vi "NamesofPMUsElements.vi"(8 "DigitalNum":u8, 9 "AnalogNum":u8, 10 "PhasorsNum":u8, 11 "data in":string) -> (1 "Phasor Digitals":i32(listbox), 2 "PMU Analogs":i32(listbox), 3 "Phasor Names":i32(listbox))   [LabVIEW 2013]
panel:
  out "DIGUNIT":string
  out "ANUNIT":string
  out "PHUNIT":string
  out "RET_DATA":T1
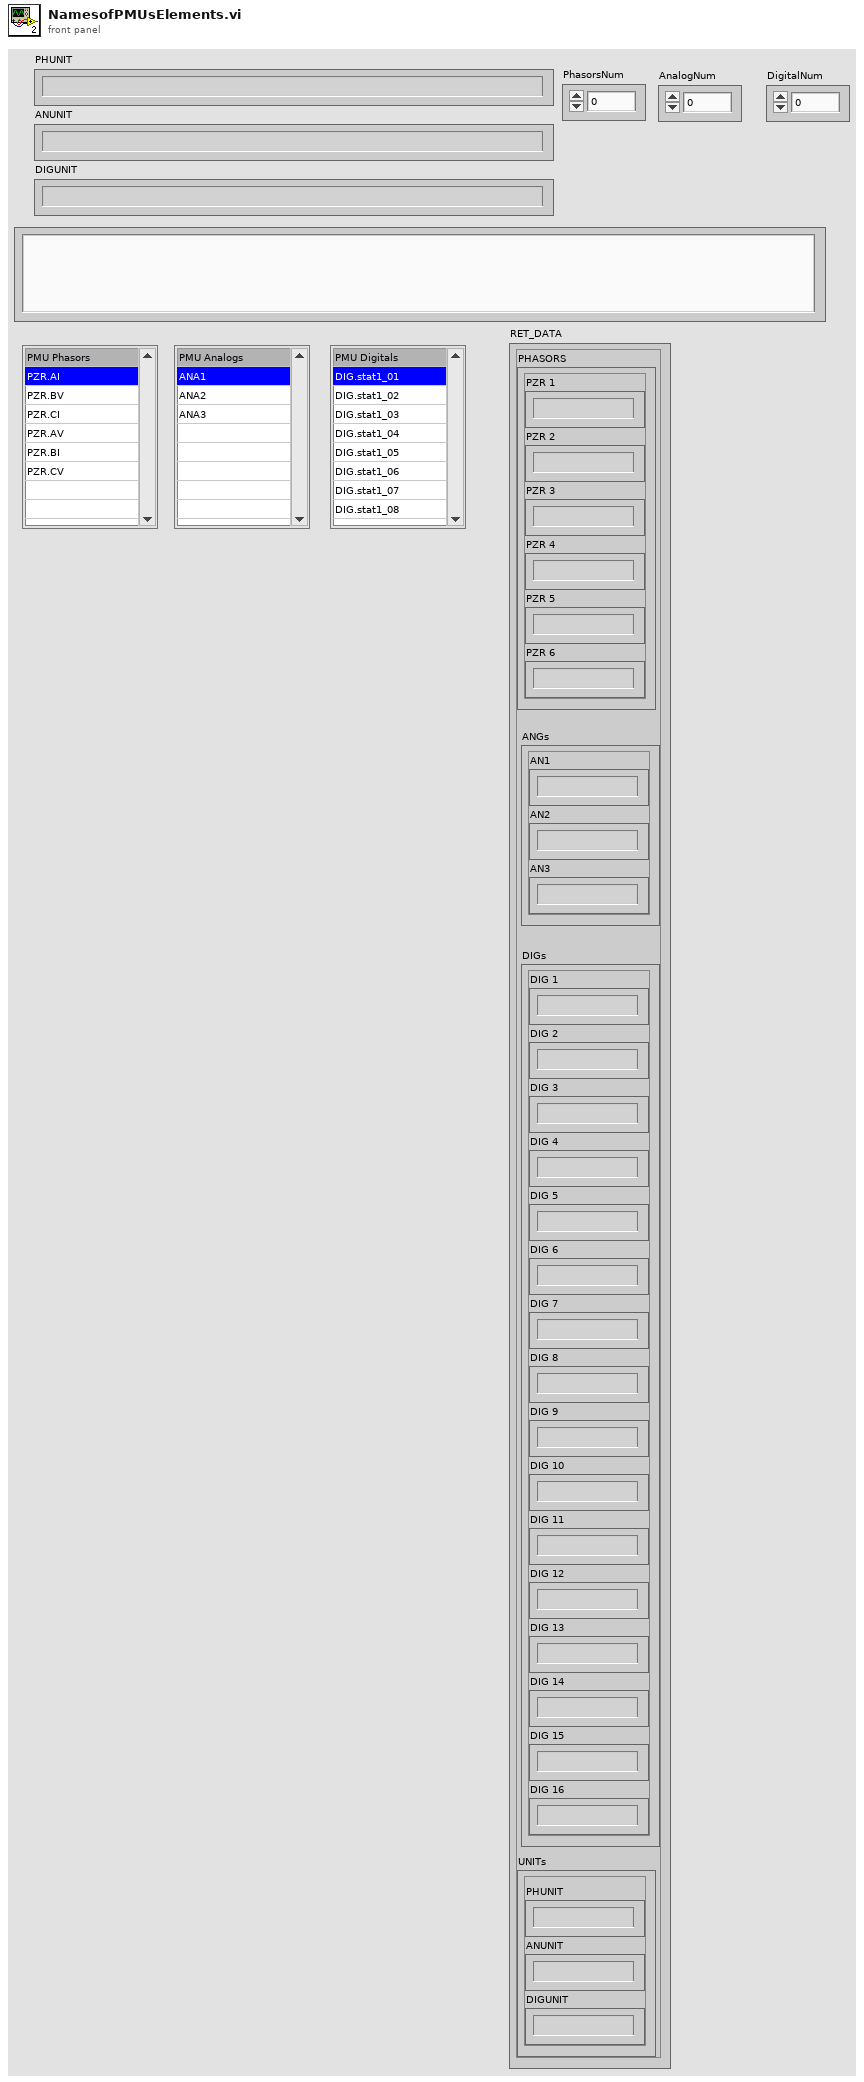
[diagram p1: front panel]
types:
  T1 = cluster{"PHASORS":cluster{"PZR 1":string, "PZR 2":string, "PZR 3":string, "PZR 4":string, "PZR 5":string, "PZR 6":string}, "ANGs":cluster{"AN1":string, "AN2":string, "AN3":string}, "DIGs":cluster{"DIG 1":string, "DIG 2":string, "DIG 3":string, "DIG 4":string, "DIG 5":string, "DIG 6":string, "DIG 7":string, "DIG 8":string, "DIG 9":string, "DIG 10":string, "DIG 11":string, "DIG 12":string, "DIG 13":string, "DIG 14":string, "DIG 15":string, "DIG 16":string}, "UNITs":cluster{"PHUNIT":string, "ANUNIT":string, "DIGUNIT":string}}
  T2 = cluster{"DIG 1":string, "DIG 2":string, "DIG 3":string, "DIG 4":string, "DIG 5":string, "DIG 6":string, "DIG 7":string, "DIG 8":string, "DIG 9":string, "DIG 10":string, "DIG 11":string, "DIG 12":string, "DIG 13":string, "DIG 14":string, "DIG 15":string, "DIG 16":string}
  T3 = cluster{"PHUNIT":string, "ANUNIT":string, "DIGUNIT":string}
  T4 = cluster{"AN1":string, "AN2":string, "AN3":string}
  T5 = cluster{"PZR 1":string, "PZR 2":string, "PZR 3":string, "PZR 4":string, "PZR 5":string, "PZR 6":string}
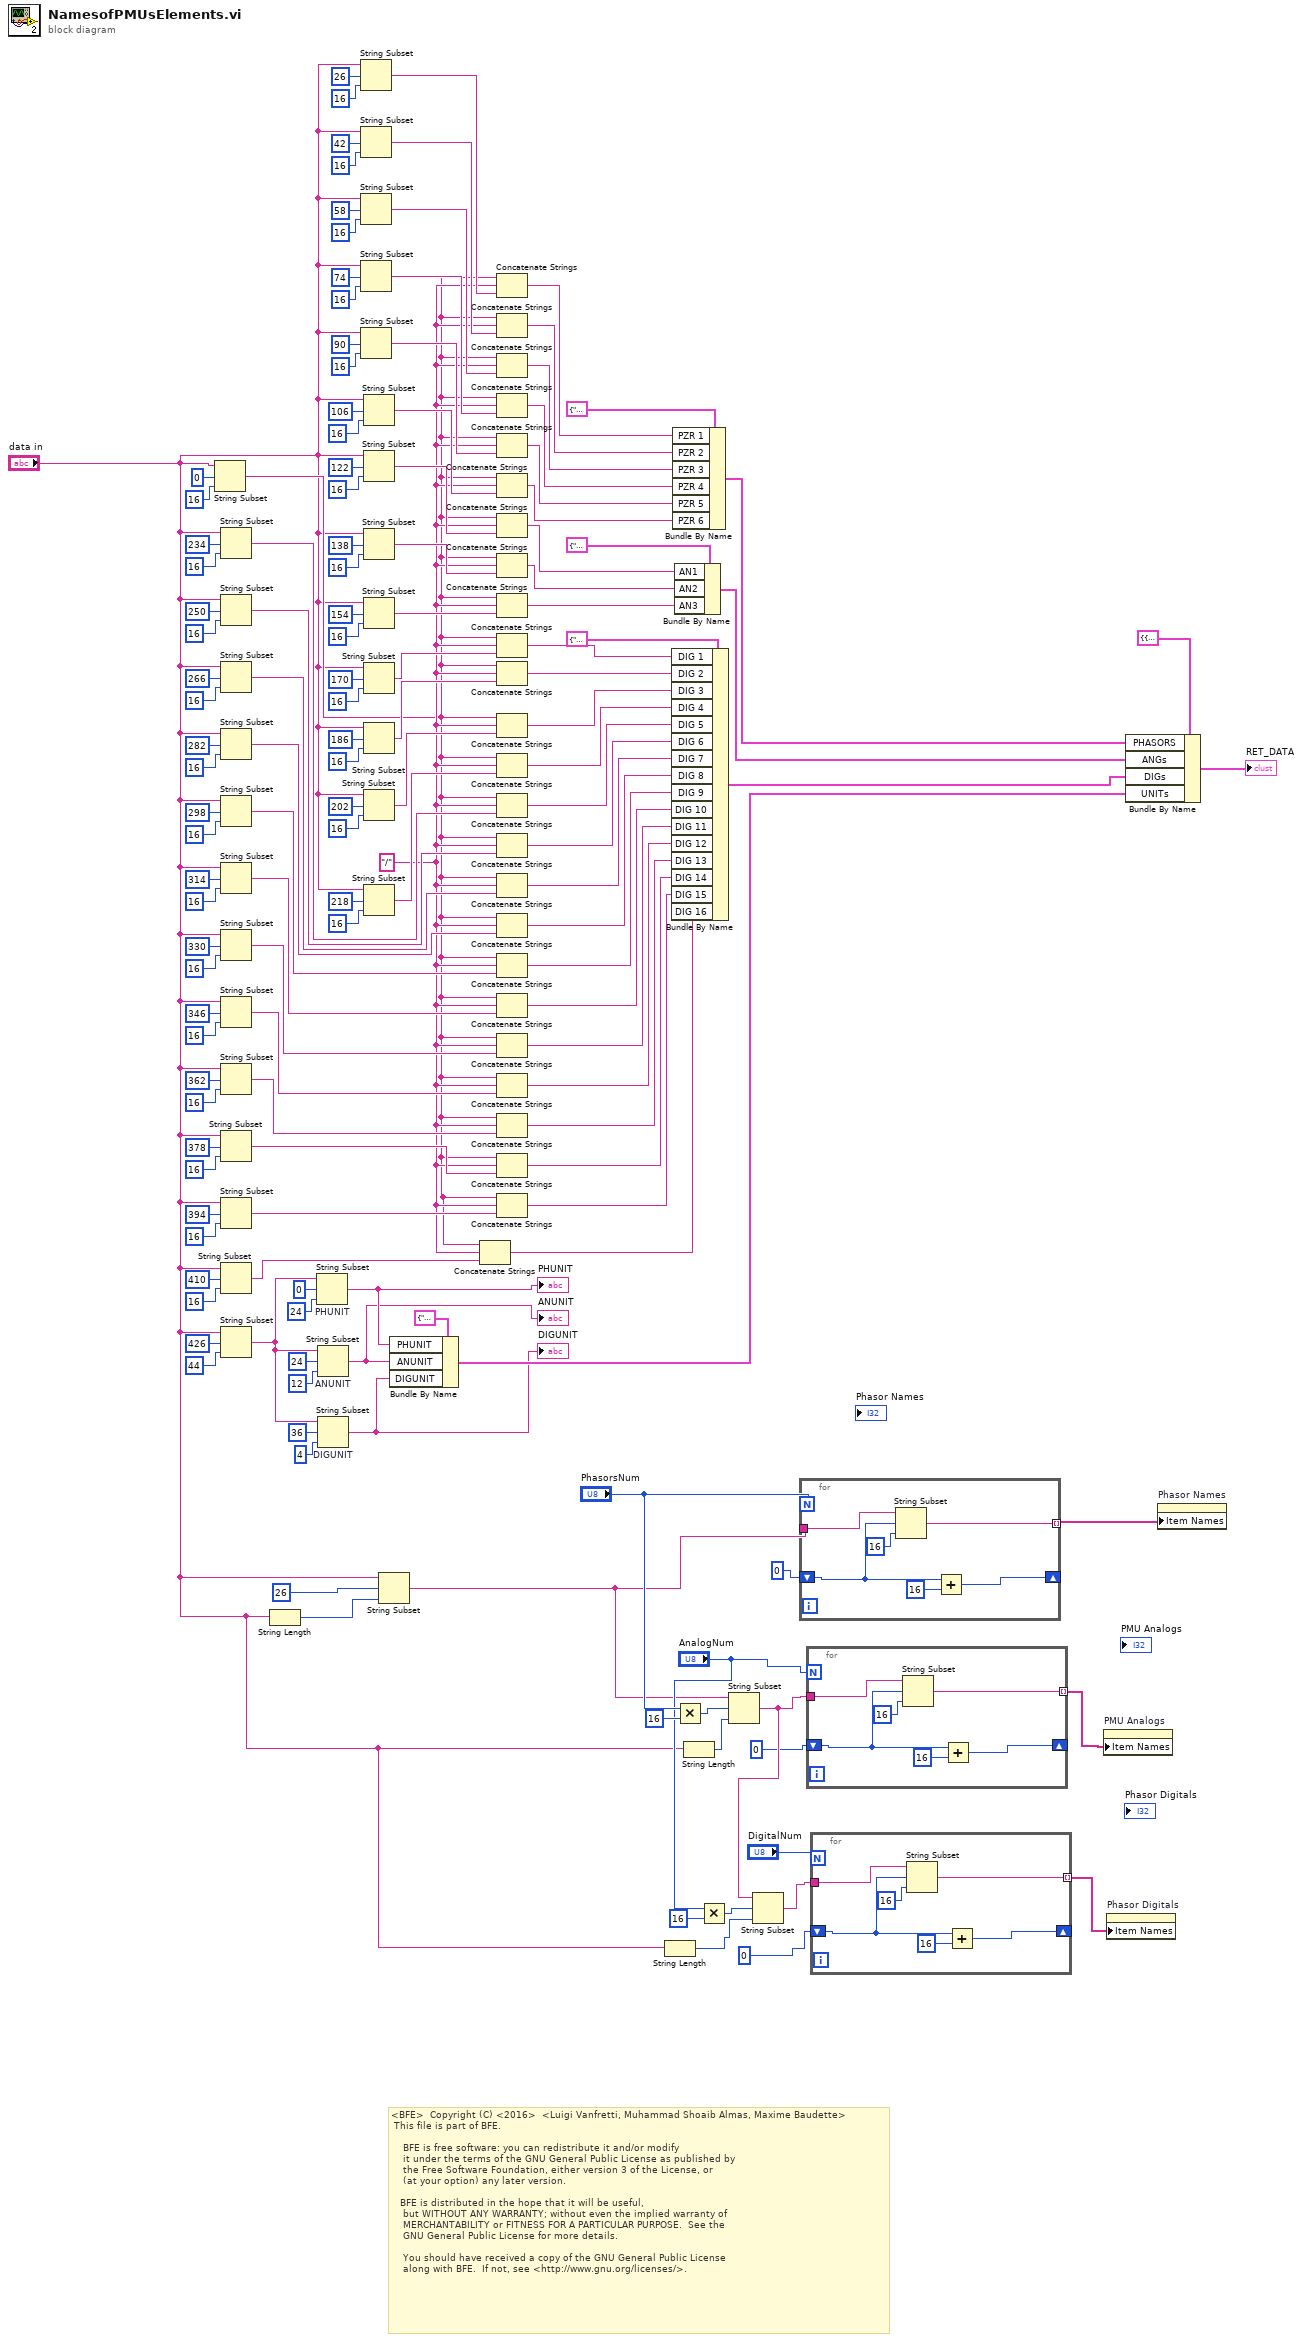
[diagram p0: block diagram]
diagram:
  w28 = "/"
  # "<BFE>  Copyright (C) <2016>  <Luigi Vanfretti, Muhammad Shoaib Almas, Maxime Baudette>\n This file is part of BFE.\n\n    BFE is free software: you can redistribute it and/or modify\n    it under the terms of the GNU General Public License as published by\n    the Free Software Foundation, either version 3 of the License, or\n    (at your option) any later version.\n\n   BFE is distributed in the hope that it will be useful,\n    but WITHOUT ANY WARRANTY; without even the implied warranty of\n    MERCHANTABILITY or FITNESS FOR A PARTICULAR PURPOSE.  See the\n    GNU General Public License for more details.\n\n    You should have received a copy of the GNU General Public License\n    along with BFE.  If not, see <http://www.gnu.org/licenses/>."
  n1 = String Subset(string="data in", offset (0)=0, length (rest)=16 ("length (rest)")) -> (substring=w27:string)
  n2 = String Subset(string="data in", offset (0)=234, length (rest)=16 ("length (rest)")) -> (substring=w79:string)
  n3 = String Subset(string="data in", offset (0)=250, length (rest)=16 ("length (rest)")) -> (substring=w80:string)
  n4 = String Subset(string="data in", offset (0)=266, length (rest)=16 ("length (rest)")) -> (substring=w81:string)
  n5 = String Subset(string="data in", offset (0)=282, length (rest)=16 ("length (rest)")) -> (substring=w82:string)
  n6 = String Subset(string="data in", offset (0)=298, length (rest)=16 ("length (rest)")) -> (substring=w83:string)
  n7 = String Subset(string="data in", offset (0)=314, length (rest)=16 ("length (rest)")) -> (substring=w84:string)
  n8 = String Subset(string="data in", offset (0)=330, length (rest)=16 ("length (rest)")) -> (substring=w85:string)
  n9 = String Subset(string="data in", offset (0)=346, length (rest)=16 ("length (rest)")) -> (substring=w86:string)
  n10 = String Subset(string="data in", offset (0)=362, length (rest)=16 ("length (rest)")) -> (substring=w87:string)
  n11 = String Subset(string="data in", offset (0)=378, length (rest)=16 ("length (rest)")) -> (substring=w88:string)
  n12 = String Subset(string="data in", offset (0)=394, length (rest)=16 ("length (rest)")) -> (substring=w44:string)
  n13 = String Subset(string="data in", offset (0)=410, length (rest)=16 ("length (rest)")) -> (substring=w29:string)
  n14 = String Subset(string="data in", offset (0)=426, length (rest)=44 ("length (rest)")) -> (substring=w33:string)
  n15 = String Length(string="data in") -> (length=w20:i32)
  n16 = String Subset "PHUNIT"(string=w33, offset (0)=0, length (rest)=24 ("length (rest)")) -> (substring=w32:string)
  "PHUNIT" <- w32
  n17 = String Subset "ANUNIT"(string=w33, offset (0)=24, length (rest)=12 ("length (rest)")) -> (substring=w30:string)
  "ANUNIT" <- w30
  n18 = String Subset "DIGUNIT"(string=w33, offset (0)=36, length (rest)=4 ("length (rest)")) -> (substring=w31:string)
  "DIGUNIT" <- w31
  n19 = String Subset(string="data in", offset (0)=26, length (rest)=16 ("length (rest)")) -> (substring=w133:string)
  n20 = String Subset(string="data in", offset (0)=42, length (rest)=16 ("length (rest)")) -> (substring=w132:string)
  n21 = String Subset(string="data in", offset (0)=58, length (rest)=16 ("length (rest)")) -> (substring=w131:string)
  n22 = String Subset(string="data in", offset (0)=74, length (rest)=16 ("length (rest)")) -> (substring=w130:string)
  n23 = String Subset(string="data in", offset (0)=90, length (rest)=16 ("length (rest)")) -> (substring=w129:string)
  n24 = String Subset(string="data in", offset (0)=106, length (rest)=16 ("length (rest)")) -> (substring=w128:string)
  n25 = String Subset(string="data in", offset (0)=122, length (rest)=16 ("length (rest)")) -> (substring=w121:string)
  n26 = String Subset(string="data in", offset (0)=138, length (rest)=16 ("length (rest)")) -> (substring=w120:string)
  n27 = String Subset(string="data in", offset (0)=154, length (rest)=16 ("length (rest)")) -> (substring=w119:string)
  n28 = String Subset(string="data in", offset (0)=170, length (rest)=16 ("length (rest)")) -> (substring=w75:string)
  n29 = String Subset(string="data in", offset (0)=186, length (rest)=16 ("length (rest)")) -> (substring=w76:string)
  n30 = String Subset(string="data in", offset (0)=202, length (rest)=16 ("length (rest)")) -> (substring=w77:string)
  n31 = String Subset(string="data in", offset (0)=218, length (rest)=16 ("length (rest)")) -> (substring=w78:string)
  n32 = String Subset(string="data in", offset (0)=26, length (rest)=w20) -> (substring=w4:string)
  n33 = Bundle By Name(cluster=T3 {"PHUNIT"="", "ANUNIT"="", "DIGUNIT"=""}, "PHUNIT"=w32, "ANUNIT"=w30, "DIGUNIT"=w31) -> (w36:T3)
  n34 = Concatenate Strings(w27, w28, w29) -> (w26:string)
  n35 = Concatenate Strings(w27, w28, w133) -> (w58:string)
  n36 = Concatenate Strings(w27, w28, w132) -> (w57:string)
  n37 = Concatenate Strings(w27, w28, w131) -> (w56:string)
  n38 = Concatenate Strings(w27, w28, w130) -> (w55:string)
  n39 = Concatenate Strings(w27, w28, w129) -> (w54:string)
  n40 = Concatenate Strings(w27, w28, w128) -> (w53:string)
  n41 = Concatenate Strings(w27, w28, w121) -> (w51:string)
  n42 = Concatenate Strings(w27, w28, w120) -> (w50:string)
  n43 = Concatenate Strings(w27, w28, w119) -> (w49:string)
  n44 = Concatenate Strings(w27, w28, w75) -> (w74:string)
  n45 = Concatenate Strings(w27, w28, w76) -> (w73:string)
  n46 = Concatenate Strings(w27, w28, w77) -> (w72:string)
  n47 = Concatenate Strings(w27, w28, w78) -> (w61:string)
  n48 = Concatenate Strings(w27, w28, w79) -> (w71:string)
  n49 = Concatenate Strings(w27, w28, w80) -> (w70:string)
  n50 = Concatenate Strings(w27, w28, w81) -> (w60:string)
  n51 = Concatenate Strings(w27, w28, w82) -> (w69:string)
  n52 = Concatenate Strings(w27, w28, w83) -> (w68:string)
  n53 = Concatenate Strings(w27, w28, w84) -> (w67:string)
  n54 = Concatenate Strings(w27, w28, w85) -> (w66:string)
  n55 = Concatenate Strings(w27, w28, w86) -> (w65:string)
  n56 = Concatenate Strings(w27, w28, w87) -> (w64:string)
  n57 = Concatenate Strings(w27, w28, w88) -> (w63:string)
  n58 = Concatenate Strings(w27, w28, w44) -> (w62:string)
  n59 = String Length(string="data in") -> (length=w3:i32)
  n60 = Bundle By Name(cluster=T2 {"DIG 1"="PMU.133/DIG.stat1_01    ", "DIG 2"="PMU.133/DIG.stat1_02    ", "DIG 3"="PMU.133/DIG.stat1_03    ", "DIG 4"="PMU.133/DIG.stat1_04    ", "DIG 5"="PMU.133/DIG.stat1_05    ", "DIG 6"="PMU.133/DIG.stat1_06    ", "DIG 7"="PMU.133/DIG.stat1_07    ", "DIG 8"="PMU.133/DIG.stat1_08    ", "DIG 9"="PMU.133/DIG.stat1_09    ", "DIG 10"="PMU.133/DIG.stat1_10    ", "DIG 11"="PMU.133/DIG.stat1_11    ", "DIG 12"="PMU.133/DIG.stat1_12    ", "DIG 13"="PMU.133/DIG.stat1_13    ", "DIG 14"="PMU.133/DIG.stat1_14    ", "DIG 15"="PMU.133/DIG.stat1_15    ", "DIG 16"="PMU.133/DIG.stat1_15    "}, "DIG 1"=w74, "DIG 2"=w73, "DIG 3"=w72, "DIG 4"=w61, "DIG 5"=w71, "DIG 6"=w70, "DIG 7"=w60, "DIG 8"=w69, "DIG 9"=w68, "DIG 10"=w67, "DIG 11"=w66, "DIG 12"=w65, "DIG 13"=w64, "DIG 14"=w63, "DIG 15"=w62, "DIG 16"=w26) -> (w23:T2)
  n61 = Bundle By Name(cluster=T5 {"PZR 1"="PMU.133/PZR.AI          ", "PZR 2"="PMU.133/PZR.BV          ", "PZR 3"="PMU.133/PZR.CI          ", "PZR 4"="PMU.133/PZR.AV          ", "PZR 5"="PMU.133/PZR.BI          ", "PZR 6"="PMU.133/PZR.CV          "}, "PZR 1"=w58, "PZR 2"=w57, "PZR 3"=w56, "PZR 4"=w55, "PZR 5"=w54, "PZR 6"=w53) -> (w25:T5)
  n62 = Bundle By Name(cluster=T4 {"AN1"="PMU.133/ANA1            ", "AN2"="PMU.133/ANA2            ", "AN3"="PMU.133/ANA3            "}, "AN1"=w51, "AN2"=w50, "AN3"=w49) -> (w24:T4)
  n63 = Multiply(x="PhasorsNum", y=u8 16) -> (x*y=w17:u8)
  n64 = String Length(string="data in") -> (length=w7:i32)
  n65 = Multiply(x="AnalogNum", y=u8 16) -> (x*y=w12:u8)
  n66 = String Subset(string=w4, offset (0)=w17, length (rest)=w7) -> (substring=w11:string)
  n67 = String Subset(string=w11, offset (0)=w12, length (rest)=w3) -> (substring=w9:string)
  n68 = for {
    N: "PhasorsNum" -> [_]
    tunnel: w4 -> [w153]
    tunnel: [w151] -> w19 mode=indexing
    shift-right: [w148] -> _
    shift-left: 0 ("offset (0)") -> [w150]
    n69 = String Subset(string=w153, offset (0)=w150, length (rest)=16 ("length (rest)")) -> (substring=w151:string)
    n70 = Add(x=w150, y=16) -> (x+y=w148:i32)
  }
  n71 = for {
    N: "AnalogNum" -> [_]
    tunnel: w11 -> [w159]
    tunnel: [w157] -> w14 mode=indexing
    shift-right: [w154] -> _
    shift-left: 0 ("offset (0)") -> [w156]
    n72 = String Subset(string=w159, offset (0)=w156, length (rest)=16 ("length (rest)")) -> (substring=w157:string)
    n73 = Add(x=w156, y=16) -> (x+y=w154:i32)
  }
  n74 = for {
    N: "DigitalNum" -> [_]
    tunnel: w9 -> [w165]
    tunnel: [w163] -> w8 mode=indexing
    shift-right: [w160] -> _
    shift-left: 0 ("offset (0)") -> [w162]
    n75 = String Subset(string=w165, offset (0)=w162, length (rest)=16 ("length (rest)")) -> (substring=w163:string)
    n76 = Add(x=w162, y=16) -> (x+y=w160:i32)
  }
  n77 = property on="PMU Analogs" class="LstBox (strict)"("Item Names"=w14) -> ()  [unwired: 2 in, 2 out]
  n78 = property on="Phasor Digitals" class="LstBox (strict)"("Item Names"=w8) -> ()  [unwired: 2 in, 2 out]
  n79 = Bundle By Name(cluster=T1 {"PHASORS"={"PZR 1"="PMU.133/PZR.AI          ", "PZR 2"="PMU.133/PZR.BV          ", "PZR 3"="PMU.133/PZR.CI          ", "PZR 4"="PMU.133/PZR.AV          ", "PZR 5"="PMU.133/PZR.BI          ", "PZR 6"="PMU.133/PZR.CV          "}, "ANGs"={"AN1"="PMU.133/ANA1            ", "AN2"="PMU.133/ANA2            ", "AN3"="PMU.133/ANA3            "}, "DIGs"={"DIG 1"="PMU.133/DIG.stat1_01    ", "DIG 2"="PMU.133/DIG.stat1_02    ", "DIG 3"="PMU.133/DIG.stat1_03    ", "DIG 4"="PMU.133/DIG.stat1_04    ", "DIG 5"="PMU.133/DIG.stat1_05    ", "DIG 6"="PMU.133/DIG.stat1_06    ", "DIG 7"="PMU.133/DIG.stat1_07    ", "DIG 8"="PMU.133/DIG.stat1_08    ", "DIG 9"="PMU.133/DIG.stat1_09    ", "DIG 10"="PMU.133/DIG.stat1_10    ", "DIG 11"="PMU.133/DIG.stat1_11    ", "DIG 12"="PMU.133/DIG.stat1_12    ", "DIG 13"="PMU.133/DIG.stat1_13    ", "DIG 14"="PMU.133/DIG.stat1_14    ", "DIG 15"="PMU.133/DIG.stat1_15    ", "DIG 16"="PMU.133/DIG.stat1_15    "}, "UNITs"={"PHUNIT"="", "ANUNIT"="", "DIGUNIT"=""}}, "PHASORS"=w25, "ANGs"=w24, "DIGs"=w23, "UNITs"=w36) -> (→"RET_DATA":T1)
  n80 = property on="Phasor Names" class="LstBox (strict)"("Item Names"=w19) -> ()  [unwired: 2 in, 2 out]
